vi "ReadIO.loop.fpga.vi"(9 "Delta time":u32, 10 "Number of time points":i32) -> ()   [LabVIEW 2012]
uses:
  <vilib>/eio/EIONode/EIONode.xnode
  <vilib>/Platform/TimedLoop/XDataNode/XDataNode.xnode
  <vilib>/Platform/TimedLoop/XDataNode/nitl_modes.ctl
  <vilib>/Platform/TimedLoop/XDataNode/XDNodeRunTimeDep.lvlib
  <vilib>/Platform/TimedLoop/XDataNode/wakeup.ctl
  <vilib>/Platform/TimedLoop/XDataNode/timing_clust.ctl
  <vilib>/rvi/eio/common/nirviEmuTemplateMethod_errors.vi
  <vilib>/rvi/DataTransferAndStorage/Container/XNode/niFpgaContainer.xnode
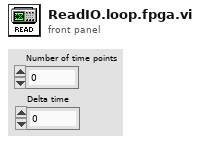
[diagram p1: front panel]
types:
  T1 = typedef "XDNodeRunTimeDep.lvlib/timing_clust.ctl" = cluster{"Expected End [f-1]":u64, "Actual End [f-1]":u64, "Finished Late? [f-1]":bool, "Expected End [i-1]":u64, "Actual End [i-1]":u64, "Finished Late? [i-1]":bool, "Expected Start [i]":u64, "Actual Start [i]":u64, "Expected Start [f]":u64, "Actual Start [f]":u64, "Source Name":string, "Structure Name":string, "Period":i64, "Deadline":i64, "Offset":i64, "Start":i64, "Priority":i32, "Timeout":i32, "Mode":T2, "Wakeup Reason":T3, "Error":errorcluster, "Source Type":string, "Secondary Source Type":string, "Global End Time":u64, "Global Start Time":u64, "Frame Duration":u64, "Iteration Duration":u64, "Assigned CPU":i32, "I/O Scan Engine Mode":u32}
  T2 = typedef "XDNodeRunTimeDep.lvlib/nitl_modes.ctl" = enum32{"No Change", "Process missed periods, maintain original phase", "Discard missed periods, maintain original phase", "Process missed periods, ignore original phase", "Discard missed periods, ignore original phase"}
  T3 = typedef "XDNodeRunTimeDep.lvlib/wakeup.ctl" = enum32{"Normal", "Aborted", "Asynchronous wakeup", "Timing source error", "Timed loop error", "Timeout"}
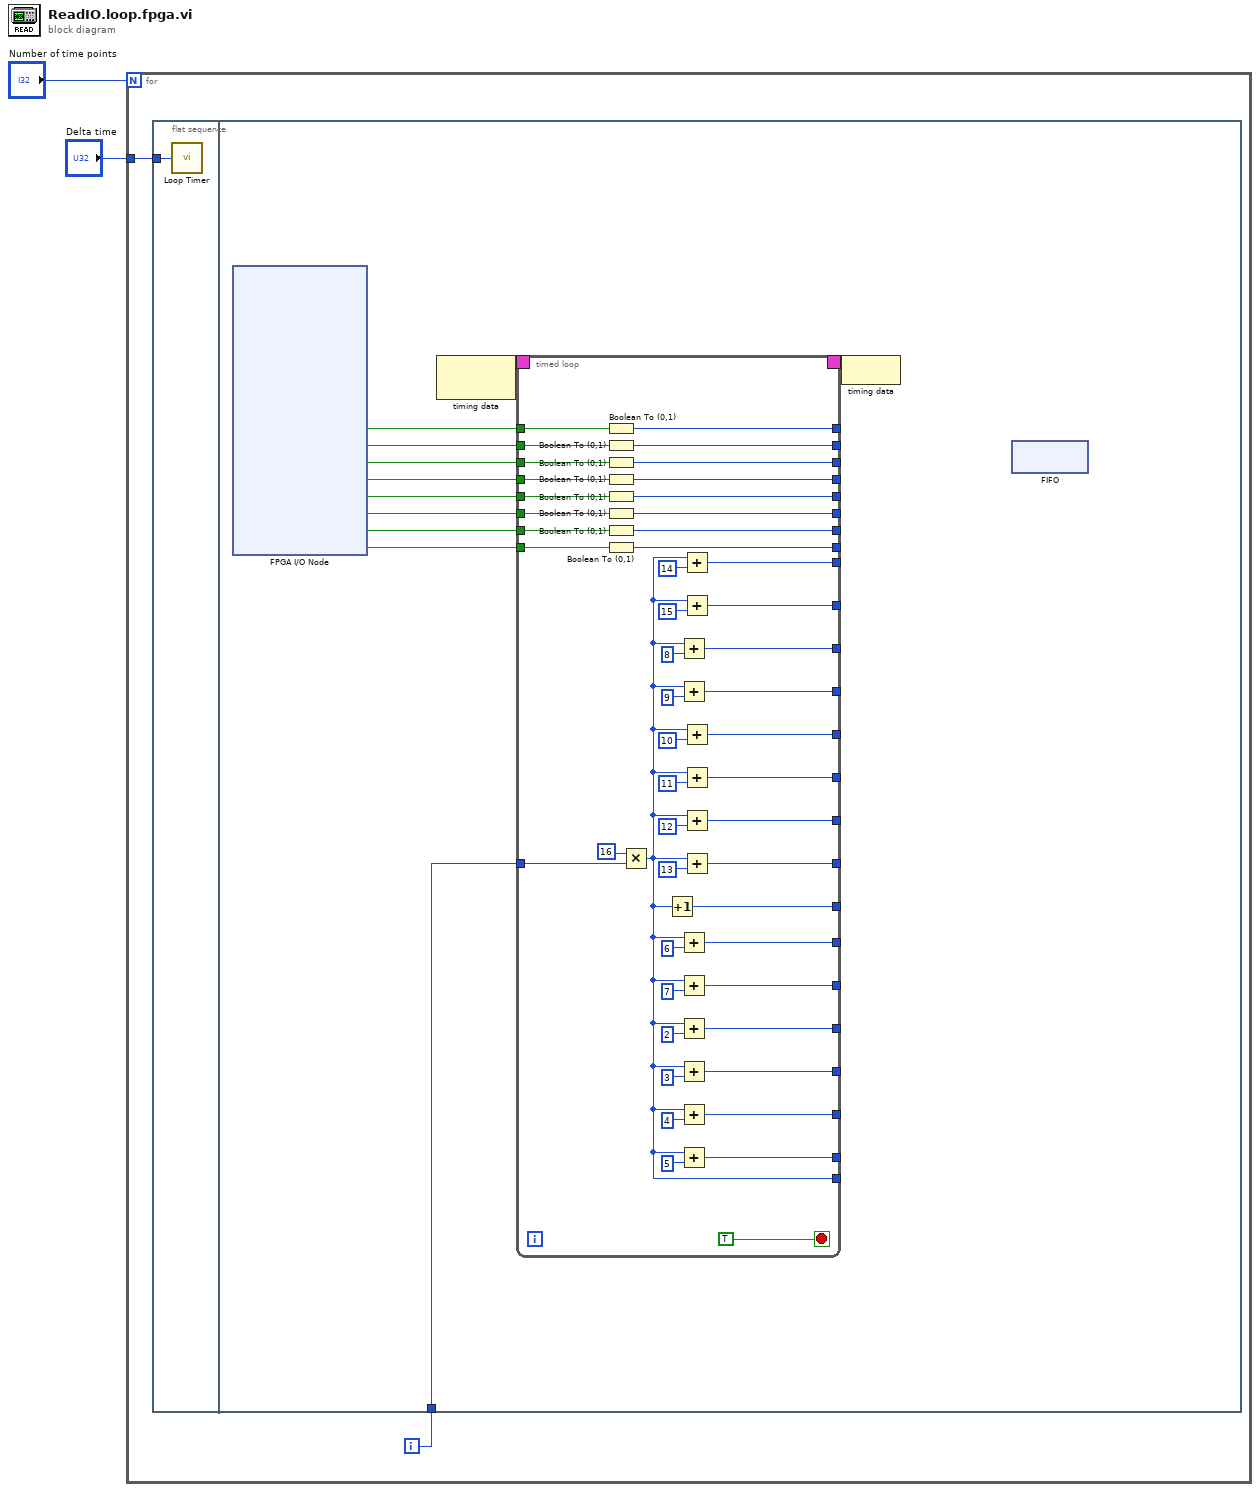
[diagram p0: block diagram]
diagram:
  n1 = for {
    N: "Number of time points" -> [_]
    tunnel: "Delta time" -> [w4]
    i -> [w3]
    n2 = flat-sequence {
      tunnel: w4 -> [w5]
      tunnel: w3 -> [w6]
      frame #0 {
        n3 = call "Loop Timer"("Count(uSec)"=w5) -> ()  [unwired: 1 out]
      }
      frame #1 {
        n4 = xnode "FPGA I/O Node"() -> ("Connector0/AI2"=w22:i16, "Connector0/AI3"=w21:i16, "Connector0/AI4"=w20:i16, "Connector0/AI5"=w19:i16, "Connector0/AI6"=w18:i16, "Connector0/AI7"=w17:i16, "Connector0/DIO8"=w16:bool, "Connector0/DIO9"=w15:bool, "Connector0/DIO10"=w14:bool, "Connector0/DIO11"=w13:bool, "Connector0/DIO12"=w12:bool, "Connector0/DIO13"=w11:bool, "Connector0/DIO14"=w10:bool, "Connector0/DIO15"=w9:bool)  [unwired: 16 in, 18 out]
        n5 = node-c288() -> (w8:T1)  [unwired: 1 in]
        n6 = timed-loop {
          timing: w8 -> [_]
          timing-out: [_] -> w7
          tunnel: w16 -> [w71]
          tunnel: w15 -> [w70]
          tunnel: w14 -> [w69]
          tunnel: w13 -> [w68]
          tunnel: w12 -> [w67]
          tunnel: w11 -> [w66]
          tunnel: w10 -> [w65]
          tunnel: w9 -> [w64]
          tunnel: [w63] -> _
          tunnel: [w61] -> _
          tunnel: [w59] -> _
          tunnel: [w57] -> _
          tunnel: [w55] -> _
          tunnel: [w53] -> _
          tunnel: [w51] -> _
          tunnel: [w49] -> _
          tunnel: [w47] -> _
          tunnel: [w45] -> _
          tunnel: [w43] -> _
          tunnel: [w41] -> _
          tunnel: [w39] -> _
          tunnel: [w38] -> _
          tunnel: [w37] -> _
          tunnel: [w36] -> _
          tunnel: [w35] -> _
          tunnel: [w34] -> _
          tunnel: [w33] -> _
          tunnel: [w31] -> _
          tunnel: [w29] -> _
          tunnel: [w28] -> _
          tunnel: [w27] -> _
          tunnel: w6 -> [w25]
          tunnel: [w23] -> _
          stop <- TRUE stop-if-true
          n7 = Boolean To (0,1)(Boolean=w71) -> (0, 1=w34:i16)
          n8 = Boolean To (0,1)(Boolean=w70) -> (0, 1=w35:i16)
          n9 = Boolean To (0,1)(Boolean=w69) -> (0, 1=w36:i16)
          n10 = Boolean To (0,1)(Boolean=w68) -> (0, 1=w37:i16)
          n11 = Boolean To (0,1)(Boolean=w67) -> (0, 1=w38:i16)
          n12 = Boolean To (0,1)(Boolean=w66) -> (0, 1=w39:i16)
          n13 = Boolean To (0,1)(Boolean=w65) -> (0, 1=w28:i16)
          n14 = Boolean To (0,1)(Boolean=w64) -> (0, 1=w27:i16)
          n15 = Multiply(x=u32 16, y=w25) -> (x*y=w23:u32)
          n16 = Increment(x=w23) -> (x+1=w33:u32)
          n17 = Add(x=w23, y=u32 8) -> (x+y=w53:u32)
          n18 = Add(x=w23, y=u32 9) -> (x+y=w55:u32)
          n19 = Add(x=w23, y=u32 6) -> (x+y=w49:u32)
          n20 = Add(x=w23, y=u32 7) -> (x+y=w51:u32)
          n21 = Add(x=w23, y=u32 2) -> (x+y=w41:u32)
          n22 = Add(x=w23, y=u32 3) -> (x+y=w43:u32)
          n23 = Add(x=w23, y=u32 4) -> (x+y=w45:u32)
          n24 = Add(x=w23, y=u32 5) -> (x+y=w47:u32)
          n25 = Add(x=w23, y=u32 14) -> (x+y=w31:u32)
          n26 = Add(x=w23, y=u32 15) -> (x+y=w29:u32)
          n27 = Add(x=w23, y=u32 10) -> (x+y=w57:u32)
          n28 = Add(x=w23, y=u32 11) -> (x+y=w59:u32)
          n29 = Add(x=w23, y=u32 12) -> (x+y=w61:u32)
          n30 = Add(x=w23, y=u32 13) -> (x+y=w63:u32)
        }
        n31 = node-c288(w7) -> ()
        n32 = xnode "FIFO "() -> ()  [unwired: 1 in, 1 out]
      }
    }
  }
